vi "Handle.vi"(8 "error in (no error)":errorcluster, 10 "Zero Timeout Message Handler in":refnum<class "Zero Timeout Message Handler.lvclass">, 11 "Message in":refnum<class "Loop Msg.lvclass">) -> (0 "error out":errorcluster, 2 "Zero Timeout Message Handler out":refnum<class "Zero Timeout Message Handler.lvclass">)   [LabVIEW 2024, in "PID Loop.lvlib" / "Loop Msg.lvclass"]
uses:
  Loop Msg.lvclass
  src/Zero Timeout Message Handler/Zero Timeout Message Handler/Zero Timeout Message Handler.lvclass
  PID Loop.lvclass
  Loop Msg.lvclass/Loop Msg.ctl
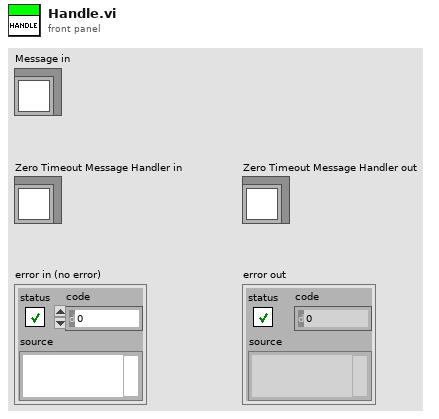
[diagram p1: front panel]
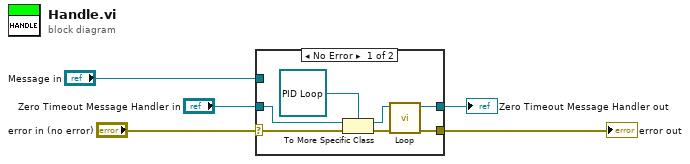
[diagram p0: block diagram]
diagram:
  n1 = case shown="No Error" "error in (no error)" {
    selector: "error in (no error)" -> [w7 w13]
    tunnel: "Zero Timeout Message Handler in" -> [w10 w14]
    tunnel: [w12 w14] -> w3
    tunnel: [w11 w13] -> w2
    tunnel: "Message in" -> [_ _]
    frame No Error {
      n2 = To More Specific Class(target class=refnum<class "PID Loop.lvclass"> refnum ("PID Loop in"), reference=w10, error in=w7) -> (specific class reference=w8:refnum<class "PID Loop.lvclass">, error out=w6:errorcluster)
      n3 = call-dynamic "Loop.vi"("error in (no error)"=w6, "PID Loop in"=w8) -> ("error out"=w11:errorcluster, "PID Loop out"=w12:refnum<class "PID Loop.lvclass">)  [unwired: 8 in]
    }
    frame Error {
    }
  }
  "error out" <- w2
  "Zero Timeout Message Handler out" <- w3
